vi "TagDB Refmgr-unRegister.vi"(8 "error in (no error)":errorcluster, 10 "Key":string, 11 "TagDB in":T1) -> (0 "error out":errorcluster, 3 "TagDB out":T1)   [LabVIEW 2017, in "TagDB RefManager.lvlib"]
uses:
  TagDB RefManager.lvlib
  <userlib>/_NEVSTOP/TagDB/Typedef/TagDB.ctl
  b82a8531-f5a8-487c-8fc1-dd96cdb734af.vi
  f708adda-48f1-4718-b054-8870cd03288c.vi
  <userlib>/_NEVSTOP/TagDB/_Support/Error/_Clear Errors.vi
  b82a8531-f5a8-487c-8fc1-dd96cdb734af.vi/29b2ea6d-6d7f-4e4a-ad31-a5cb760462c7.vi
  <userlib>/_NEVSTOP/TagDB/API/TagDB-Status.vi
  f708adda-48f1-4718-b054-8870cd03288c.vi/29b2ea6d-6d7f-4e4a-ad31-a5cb760462c7.vi
  <userlib>/_NEVSTOP/TagDB/_Support/DataAccess/_NameCacher.vi
  <userlib>/_NEVSTOP/TagDB/_Support/Error/_[error50001]Can't Found Value.vi
  <userlib>/_NEVSTOP/TagDB/_Support/Change Detector/TagDB dbChanged.vi
  <userlib>/_NEVSTOP/TagDB/_Support/DataAccess/TagDB Ref to DVR.vi
  <userlib>/_NEVSTOP/TagDB/_Support/Error/_[error50000]Invalid DB REF.vi
  <userlib>/_NEVSTOP/TagDB/_Support/URL/TRIM-BOTH-SPACE.vi
  <userlib>/_NEVSTOP/TagDB/_Support/Error/_[error50002]Invalid DataType.vi
  <vilib>/Utility/error.llb/Trim Whitespace.vi
  <userlib>/_NEVSTOP/TagDB/_Support/Error/_Build Error Cluster.vi
  <userlib>/_NEVSTOP/TagDB/TagDB.lvlib
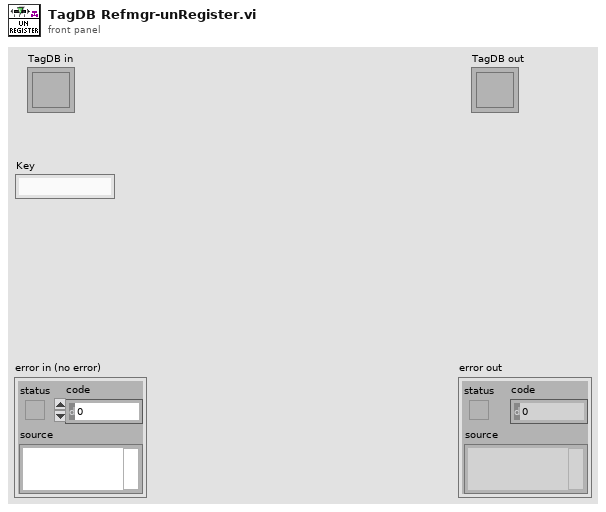
[diagram p1: front panel]
types:
  T1 = typedef "TagDB.lvlib/TagDB.ctl" = refnum<k1>
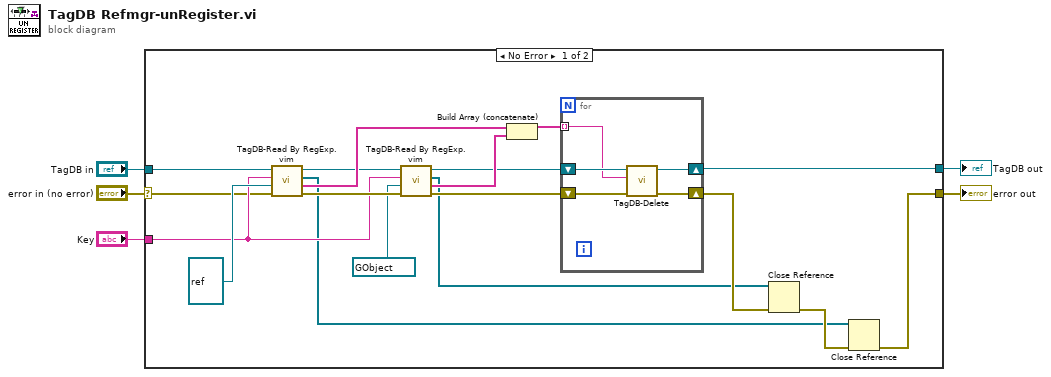
[diagram p0: block diagram]
diagram:
  n1 = case shown="No Error" "error in (no error)" {
    selector: "error in (no error)" -> [w12 w30]
    tunnel: [w23 w30] -> w4
    tunnel: [w10 w29] -> w2
    tunnel: "TagDB in" -> [w13 w29]
    tunnel: "Key" -> [w17 _]
    frame No Error {
      n2 = call "TagDB-Read By RegExp.vim"("error in (no error)"=w12, "Type"=refnum<vi> refnum ("VI out"), "RegExp"=w17, "DB Ref"=w13) -> ("error out"=w19:errorcluster, "names"=w22:string[], "value"=w6:refnum<vi>[], "DB Ref(dup)"=w20:T1)  [unwired: 4 in]
      n3 = call "TagDB-Read By RegExp.vim"("error in (no error)"=w19, "Type"=refnum<vi> refnum, "RegExp"=w17, "DB Ref"=w20) -> ("error out"=w18:errorcluster, "names"=w14:string[], "value"=w7:refnum<vi>[], "DB Ref(dup)"=w11:T1)  [unwired: 4 in]
      n4 = Build Array (concatenate)(w22, w14) -> (w15:string[])
      n5 = for {
        tunnel: w15 -> [w24] mode=indexing
        shift-right: [w27] -> w10
        shift-left: w11 -> [w28]
        shift-right: [w26] -> w8
        shift-left: w18 -> [w25]
        n6 = call <userlib>:"TagDB-Delete.vi"("error in (no error)"=w25, "name"=w24, "TagDB"=w28) -> ("error out"=w26:errorcluster, "TagDB(dup)"=w27:T1)  [unwired: 7 in]
      }
      n7 = Close Reference(reference=w7, error in (no error)=w8) -> (error out=w9:errorcluster)
      n8 = Close Reference(reference=w6, error in (no error)=w9) -> (error out=w23:errorcluster)
    }
    frame Error {
    }
  }
  "error out" <- w4
  "TagDB out" <- w2
